vi "Add Empty States to Queue Performance Test.vi"() -> ()   [LabVIEW 2013]
panel:
  out "% Improvement":dbl format="%#.1f"
  out "New":u32
  out "Old":u32
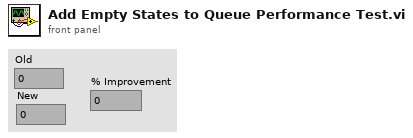
[diagram p1: front panel]
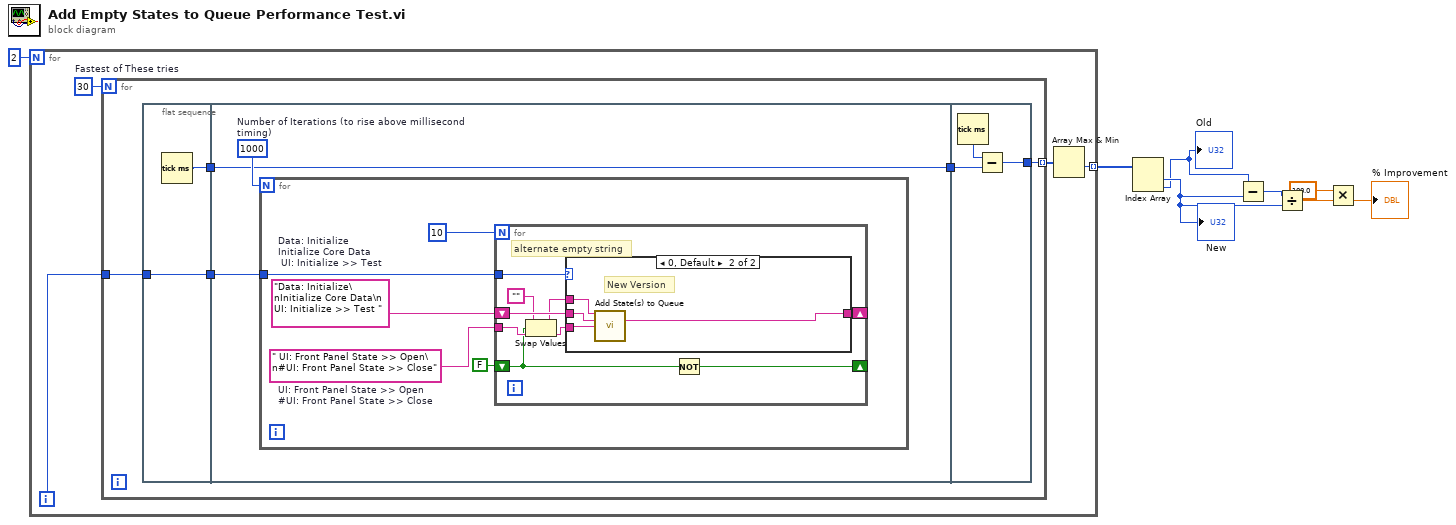
[diagram p0: block diagram]
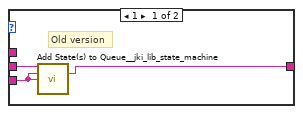
[diagram p2: hidden frame]
diagram:
  n1 = for {
    N: 2 -> [_]
    tunnel: [w9] -> w7 mode=indexing
    i -> [w12]
    w10 = 30  # Fastest of These tries
    n2 = for {
      N: w10 -> [_]
      tunnel: w12 -> [w14]
      tunnel: [w13] -> w11 mode=indexing
      n3 = flat-sequence {
        tunnel: [w19] -> w17
        tunnel: w14 -> [w18]
        tunnel: [w18] -> w16
        tunnel: w17 -> [w21]
        tunnel: [w21] -> w15
        tunnel: w16 -> [w20]
        tunnel: w15 -> [w45]
        tunnel: [w44] -> w13
        frame #0 {
          n4 = Tick Count (ms)() -> (millisecond timer value=w19:u32)
        }
        frame #1 {
          w22 = 1000  # Number of Iterations (to rise above millisecond timing)
          n5 = for {
            N: w22 -> [_]
            tunnel: w20 -> [w26]
            w24 = " UI: Front Panel State >> Open\n#UI: Front Panel State >> Close"  # UI: Front Panel State >> Open #UI: Front Panel State >> Close
            w27 = "Data: Initialize\nInitialize Core Data\n UI: Initialize >> Test "  # Data: Initialize Initialize Core Data  UI: Initialize >> Test
            n6 = for {
              N: 10 ("Numeric") -> [_]
              shift-right: [w35] -> _
              shift-left: w27 -> [w36]
              tunnel: w26 -> [w34]
              tunnel: w24 -> [w31]
              shift-right: [w28] -> _
              shift-left: FALSE -> [w29]
              # "alternate empty string"
              n7 = Swap Values(12:"", 13:w29, 14:w31) -> (1:w32:string, 3:w30:string)
              n8 = case shown="0, Default" w34 {
                tunnel: w36 -> [w39 w41]
                tunnel: [w38 w43] -> w35
                tunnel: w30 -> [w37 w42]
                tunnel: w32 -> [_ w40]
                frame 1 {
                  # "Old version"
                  n9 = call <vilib>:"Add State(s) to Queue__jki_lib_state_machine.vi"("State(s) in Front (\"\")"=w39, "State(s) in (\"\")"=w37, "State(s) at Back (\"\")"=w37) -> ("States Out"=w38:string)  [unwired: 12 in]
                }
                frame 0, Default {
                  # "New Version"
                  n10 = call "Add State(s) to Queue.vi"("State(s) in Front (\"\")"=w40, "State(s) in (\"\")"=w41, "State(s) at Back (\"\")"=w42) -> ("States Out"=w43:string)  [unwired: 12 in]
                }
              }
              n11 = Not(x=w29) -> (.not. x?=w28:bool)
            }
          }
        }
        frame #2 {
          n12 = Tick Count (ms)() -> (millisecond timer value=w46:u32)
          n13 = Subtract(x=w46, y=w45) -> (x-y=w44:u32)
        }
      }
    }
    n14 = Array Max & Min(array=w11) -> (min value=w9:u32)  [unwired: 3 out]
  }
  n15 = Index Array(array=w7) -> (element #1=w2:u32, element #2=w1:u32)  [unwired: 2 in]
  "Old" <- w1
  "New" <- w2
  n16 = Subtract(x=w1, y=w2) -> (x-y=w6:u32)
  n17 = Divide(x=w6, y=w2) -> (x/y=w5:dbl)
  n18 = Multiply(x=100.0, y=w5) -> (x*y=→"% Improvement":dbl)
